vi "数据全参数一起发送整点触发.vi"(6 "数据发送通道":enum16{"TCP", "VISA"}(ring), 8 "PW":string, 9 "MN":string) -> ()   [LabVIEW 2016, in "数据传输系统-05.lvlib"]
panel:
  out "table":string="提取小时数据"
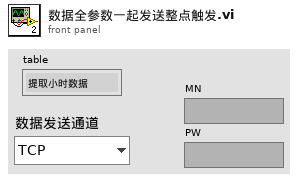
[diagram p1: front panel]
types:
  T1 = typedef "LVDateTimeRec.ctl" = cluster{"秒数的小数部分":dbl, "秒":i32, "分":i32, "时":i32, "日":i32, "月":i32, "年":i32, "天数（周）":i32, "天数（年）":i32, "DST":i32}
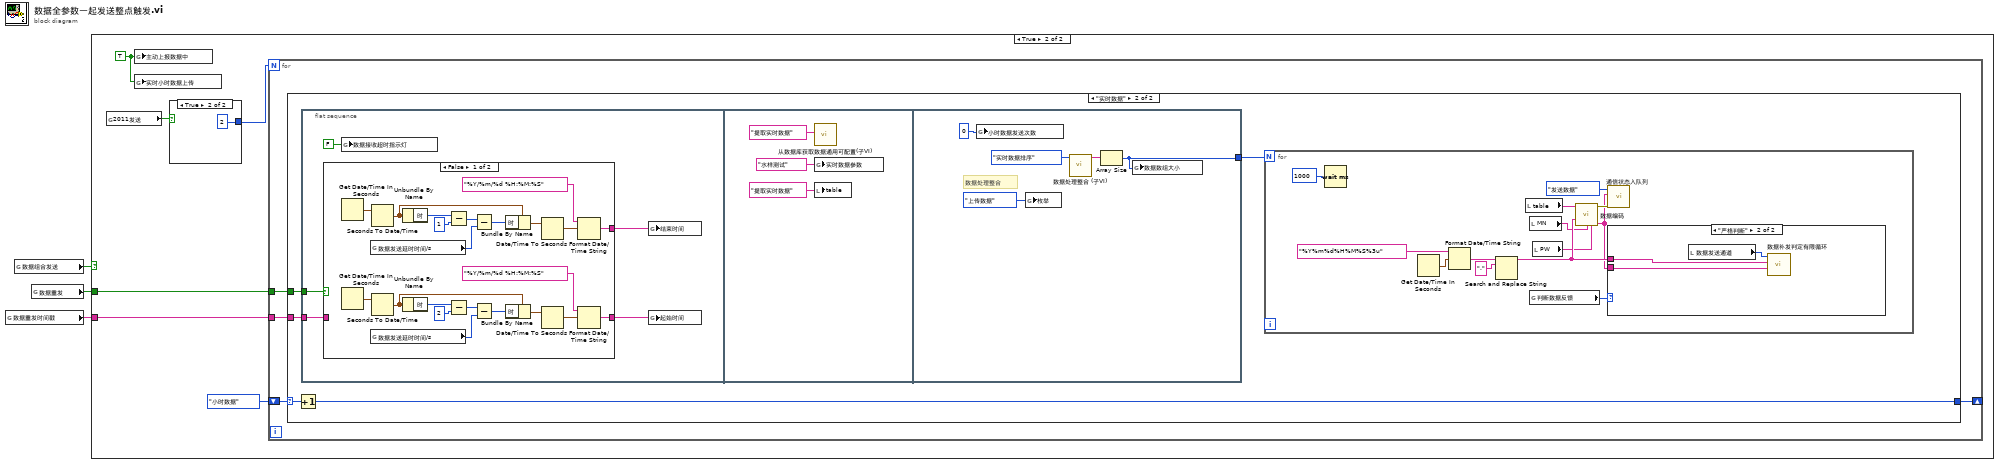
[diagram p0: block diagram]
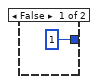
[diagram p3: hidden frame]
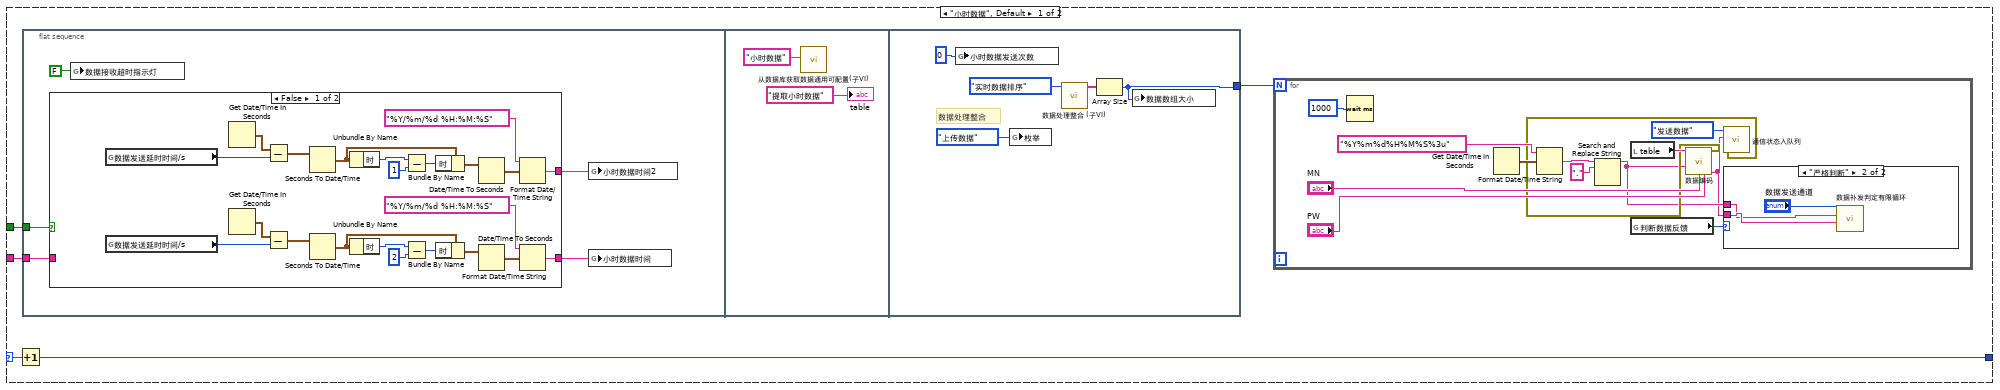
[diagram p4: hidden frame]
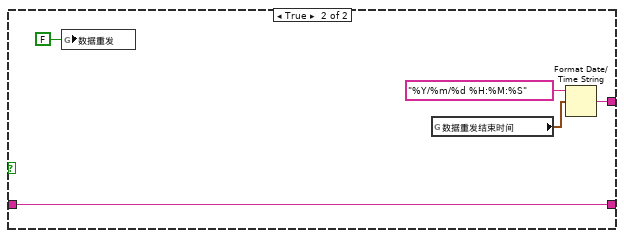
[diagram p5: hidden frame]
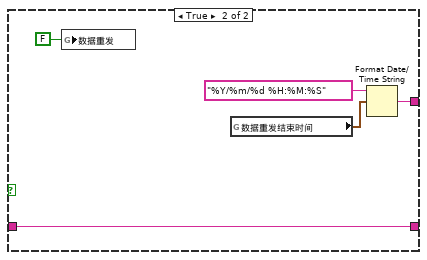
[diagram p7: hidden frame]
diagram:
  n1 = global read "断电保存全局.vi" "数据重发时间戳"() -> (w1:string)
  n2 = global read "断电保存全局.vi" "数据组合发送"() -> (w3:bool)
  n3 = global read "断电保存全局.vi" "数据重发"() -> (w2:bool)
  n4 = case shown="True" w3 {
    tunnel: w2 -> [_ w6]
    tunnel: w1 -> [_ w5]
    frame False {
    }
    frame True {
      w9 = TRUE ("主动上报数据中")
      n5 = global read "断电保存全局.vi" "2011发送"() -> (w4:bool)
      n6 = global write "全局 数据发送重叠.vi" "主动上报数据中"(w9) -> ()
      n7 = global write "全局1.vi" "实时小时数据上传"(w9) -> ()
      n8 = case shown="True" w4 {
        tunnel: [1 2] -> w7
        frame False {
        }
        frame True {
        }
      }
      n9 = for {
        N: w7 -> [_]
        shift-right: [w14] -> _
        shift-left: enum16{"小时数据", "实时数据"}."小时数据" -> [w15]
        tunnel: w6 -> [w13]
        tunnel: w5 -> [w12]
        n10 = case shown="\"实时数据\"" w15 {
          selector: w15 -> [w19 w79]
          tunnel: [w18 w78] -> w14
          tunnel: w13 -> [w17 w77]
          tunnel: w12 -> [w16 w76]
          frame "小时数据", Default {
            n11 = Increment(x=w19) -> (x+1=w18:enum16{"小时数据", "实时数据"})
            n12 = flat-sequence {
              tunnel: w17 -> [w22]
              tunnel: w16 -> [w21]
              tunnel: [w55] -> w20
              frame #0 {
                n13 = case shown="False" w22 {
                  tunnel: [w42 w52] -> w24
                  tunnel: w21 -> [_ w52]
                  tunnel: [w35 w48] -> w23
                  frame False {
                    n14 = global read "断电保存全局.vi" "数据发送延时时间/s"() -> (w27:i32)
                    n15 = global read "断电保存全局.vi" "数据发送延时时间/s"() -> (w31:i32)
                    n16 = Get Date/Time In Seconds() -> (seconds since 1Jan1904=w28:timestamp)
                    n17 = Get Date/Time In Seconds() -> (seconds since 1Jan1904=w32:timestamp)
                    n18 = Subtract(x=w28, y=w27) -> (x-y=w26:timestamp)
                    n19 = Subtract(x=w32, y=w31) -> (x-y=w30:timestamp)
                    n20 = Seconds To Date/Time(time stamp (now)=w26) -> (date time rec=w40:T1)  [unwired: 1 in]
                    n21 = Seconds To Date/Time(time stamp (now)=w30) -> (date time rec=w45:T1)  [unwired: 1 in]
                    n22 = Unbundle By Name(w40) -> ("时"=w38:i32)
                    n23 = Unbundle By Name(w45) -> ("时"=w43:i32)
                    n24 = Subtract(x=w38, y=1) -> (x-y=w29:i32)
                    n25 = Subtract(x=w43, y=2) -> (x-y=w34:i32)
                    n26 = Bundle By Name(cluster=w40, "时"=w29) -> (w41:T1)
                    n27 = Bundle By Name(cluster=w45, "时"=w34) -> (w33:T1)
                    n28 = Date/Time To Seconds(2:w41) -> (0:w36:timestamp)  [unwired: 1 in]
                    n29 = Date/Time To Seconds(2:w33) -> (0:w46:timestamp)  [unwired: 1 in]
                    n30 = Format Date/Time String(time format string (%c)="%Y/%m/%d %H:%M:%S" ("时间格式字符串(%c)"), seconds (now)=w36) -> (date/time string=w35:string)  [unwired: 1 in]
                    n31 = Format Date/Time String(time format string (%c)="%Y/%m/%d %H:%M:%S" ("时间格式字符串(%c)"), seconds (now)=w46) -> (date/time string=w42:string)  [unwired: 1 in]
                  }
                  frame True {
                    n32 = global write "断电保存全局.vi" "数据重发"(FALSE ("数据重发")) -> ()
                    n33 = global read "断电保存全局.vi" "数据重发结束时间"() -> (w50:timestamp)
                    n34 = Format Date/Time String(time format string (%c)="%Y/%m/%d %H:%M:%S" ("时间格式字符串(%c)"), seconds (now)=w50) -> (date/time string=w48:string)  [unwired: 1 in]
                  }
                }
                n35 = global write "全局 数据发送重叠.vi" "数据接收超时指示灯"(FALSE ("数据接收超时指示灯")) -> ()
                n36 = global write "全局 时间2.vi" "小时数据时间2"(w23) -> ()
                n37 = global write "全局 水样时间.vi" "小时数据时间"(w24) -> ()
              }
              frame #1 {
                n38 = call "从数据库获取数据通用可配置(子VI).vi"("table输入"="小时数据" ("名称（未命名）")) -> ()  [unwired: 9 in, 2 out]
                "table" <- "提取小时数据" ("新元素/子数组")
              }
              frame #2 {
                # "数据处理整合"
                n39 = global write "全局 小时数据发送次数.vi" "小时数据发送次数"(0 ("数值")) -> ()
                n40 = global write "全局1.vi" "枚举"(enum16{"返回请求应答", "上传数据", "返回执行结果"}."上传数据" ("枚举")) -> ()
                n41 = call "数据处理整合 (子VI).vi"("枚举"=enum16{"实时数据排序", "小时数据排序"}."实时数据排序") -> ("已排序的数组"=w56:string[])  [unwired: 10 in]
                n42 = Array Size(array=w56) -> (size(s)=w55:i32)
                n43 = global write "全局 数据数组大小.vi" "数据数组大小"(w55) -> ()
              }
            }
            n44 = for {
              N: w20 -> [_]
              n45 = Wait (ms)(milliseconds to wait=u32 1000 ("等待时间（毫秒）")) -> ()  [unwired: 1 out]
              n46 = Get Date/Time In Seconds() -> (seconds since 1Jan1904=w66:timestamp)
              n47 = Format Date/Time String(time format string (%c)="%Y%m%d%H%M%S%3u" ("时间格式字符串(%c)"), seconds (now)=w66) -> (date/time string=w67:string)  [unwired: 1 in]
              n48 = Search and Replace String(input string=w67, search string="." ("搜索字符串")) -> (result string=w62:string)  [unwired: 6 in, 3 out]
              n49 = local read "table"() -> (w72:string)
              n50 = global read "断电保存全局.vi" "判断数据反馈"() -> (w64:enum16{"非严格判断", "严格判断", "不判断"})
              n51 = call "数据编码.vi"("table输入"=w72, "QN"=w62, "MN"="MN", "PW"="PW") -> ("错误常量"=w63:errorcluster, "通讯包字符串"=w60:string)  [unwired: 10 in]
              n52 = call "通信状态入队列.vi"("错误输入（无错误）"=w63, "发送报文"=w60, "枚举"=enum16{"打开连接", "发送数据", "读取数据", "数据处理", "关闭连接"}."发送数据") -> ()  [unwired: 8 in, 1 out]
              n53 = case shown="\"严格判断\"" w64 {
                tunnel: w60 -> [_ w75]
                tunnel: w62 -> [_ w73]
                frame "非严格判断", Default {
                }
                frame "严格判断" {
                  n54 = call "数据补发判定有限循环.vi"("数据输入"=w75, "QN"=w73, "数据发送通道"="数据发送通道") -> ()  [unwired: 8 in, 1 out]
                }
              }
            }
          }
          frame "实时数据" {
            n55 = Increment(x=w79) -> (x+1=w78:enum16{"小时数据", "实时数据"})
            n56 = flat-sequence {
              tunnel: w77 -> [w84]
              tunnel: w76 -> [w83]
              tunnel: [w116] -> w80
              frame #0 {
                n57 = case shown="False" w84 {
                  tunnel: [w101 w112] -> w82
                  tunnel: w83 -> [_ w112]
                  tunnel: [w86 w108] -> w81
                  frame False {
                    n58 = Get Date/Time In Seconds() -> (seconds since 1Jan1904=w90:timestamp)
                    n59 = Get Date/Time In Seconds() -> (seconds since 1Jan1904=w97:timestamp)
                    n60 = global read "断电保存全局.vi" "数据发送延时时间/s"() -> (w89:i32)
                    n61 = global read "断电保存全局.vi" "数据发送延时时间/s"() -> (w100:i32)
                    n62 = Seconds To Date/Time(time stamp (now)=w90) -> (date time rec=w95:T1)  [unwired: 1 in]
                    n63 = Seconds To Date/Time(time stamp (now)=w97) -> (date time rec=w104:T1)  [unwired: 1 in]
                    n64 = Unbundle By Name(w95) -> ("时"=w93:i32)
                    n65 = Unbundle By Name(w104) -> ("时"=w102:i32)
                    n66 = Subtract(x=w93, y=1) -> (x-y=w88:i32)
                    n67 = Subtract(x=w102, y=2) -> (x-y=w99:i32)
                    n68 = Subtract(x=w88, y=w89) -> (x-y=w87:i32)
                    n69 = Subtract(x=w99, y=w100) -> (x-y=w98:i32)
                    n70 = Bundle By Name(cluster=w95, "时"=w87) -> (w96:T1)
                    n71 = Bundle By Name(cluster=w104, "时"=w98) -> (w105:T1)
                    n72 = Date/Time To Seconds(2:w96) -> (0:w91:timestamp)  [unwired: 1 in]
                    n73 = Date/Time To Seconds(2:w105) -> (0:w106:timestamp)  [unwired: 1 in]
                    n74 = Format Date/Time String(time format string (%c)="%Y/%m/%d %H:%M:%S" ("时间格式字符串(%c)"), seconds (now)=w91) -> (date/time string=w86:string)  [unwired: 1 in]
                    n75 = Format Date/Time String(time format string (%c)="%Y/%m/%d %H:%M:%S" ("时间格式字符串(%c)"), seconds (now)=w106) -> (date/time string=w101:string)  [unwired: 1 in]
                  }
                  frame True {
                    n76 = global write "断电保存全局.vi" "数据重发"(FALSE ("数据重发")) -> ()
                    n77 = global read "断电保存全局.vi" "数据重发结束时间"() -> (w110:timestamp)
                    n78 = Format Date/Time String(time format string (%c)="%Y/%m/%d %H:%M:%S" ("时间格式字符串(%c)"), seconds (now)=w110) -> (date/time string=w108:string)  [unwired: 1 in]
                  }
                }
                n79 = global write "全局 数据发送重叠.vi" "数据接收超时指示灯"(FALSE ("数据接收超时指示灯")) -> ()
                n80 = global write "起始时间.vi" "结束时间"(w81) -> ()
                n81 = global write "起始时间.vi" "起始时间"(w82) -> ()
              }
              frame #1 {
                n82 = call "从数据库获取数据通用可配置(子VI).vi"("table输入"="提取实时数据" ("名称（未命名）")) -> ()  [unwired: 9 in, 2 out]
                n83 = global write "全局 实时数据参数.vi" "实时数据参数"("水样测试" ("实时数据参数")) -> ()
                n84 = local write "table"("提取实时数据" ("新元素/子数组")) -> ()
              }
              frame #2 {
                # "数据处理整合"
                n85 = global write "全局 小时数据发送次数.vi" "小时数据发送次数"(0 ("数值")) -> ()
                n86 = global write "全局1.vi" "枚举"(enum16{"返回请求应答", "上传数据", "返回执行结果"}."上传数据" ("枚举")) -> ()
                n87 = call "数据处理整合 (子VI).vi"("枚举"=enum16{"实时数据排序", "小时数据排序"}."实时数据排序") -> ("已排序的数组"=w117:string[])  [unwired: 10 in]
                n88 = Array Size(array=w117) -> (size(s)=w116:i32)
                n89 = global write "全局 数据数组大小.vi" "数据数组大小"(w116) -> ()
              }
            }
            n90 = for {
              N: w80 -> [_]
              n91 = Wait (ms)(milliseconds to wait=u32 1000 ("等待时间（毫秒）")) -> ()  [unwired: 1 out]
              n92 = Get Date/Time In Seconds() -> (seconds since 1Jan1904=w129:timestamp)
              n93 = Format Date/Time String(time format string (%c)="%Y%m%d%H%M%S%3u" ("时间格式字符串(%c)"), seconds (now)=w129) -> (date/time string=w130:string)  [unwired: 1 in]
              n94 = Search and Replace String(input string=w130, search string="." ("搜索字符串")) -> (result string=w125:string)  [unwired: 6 in, 3 out]
              n95 = local read "table"() -> (w133:string)
              n96 = local read "MN"() -> (w124:string)
              n97 = global read "断电保存全局.vi" "判断数据反馈"() -> (w127:enum16{"非严格判断", "严格判断", "不判断"})
              n98 = local read "PW"() -> (w123:string)
              n99 = call "数据编码.vi"("table输入"=w133, "QN"=w125, "MN"=w124, "PW"=w123) -> ("错误常量"=w126:errorcluster, "通讯包字符串"=w121:string)  [unwired: 10 in]
              n100 = call "通信状态入队列.vi"("错误输入（无错误）"=w126, "发送报文"=w121, "枚举"=enum16{"打开连接", "发送数据", "读取数据", "数据处理", "关闭连接"}."发送数据") -> ()  [unwired: 8 in, 1 out]
              n101 = case shown="\"严格判断\"" w127 {
                tunnel: w121 -> [_ w136]
                tunnel: w125 -> [_ w135]
                frame "非严格判断", Default {
                }
                frame "严格判断" {
                  n102 = local read "数据发送通道"() -> (w134:enum16{"TCP", "VISA"})
                  n103 = call "数据补发判定有限循环.vi"("数据输入"=w136, "QN"=w135, "数据发送通道"=w134) -> ()  [unwired: 8 in, 1 out]
                }
              }
            }
          }
        }
      }
    }
  }
